vi "Open.vi"(8 "Error In":errorcluster, 10 "Username":string, 11 "Hostname / IP":string="localhost") -> (0 "Error Out":errorcluster, 3 "Hue Config":T1)   [LabVIEW 2020, in "LMH-Hue.lvlib"]
uses:
  LMH-Hue.lvlib
  Private/Type Defs/Hue Ref.ctl
  <vilib>/httpClient/ClientHandle.ctl
  Private/Type Defs/Light Data.ctl
  <vilib>/httpClient/LabVIEWHTTPClient.lvlib
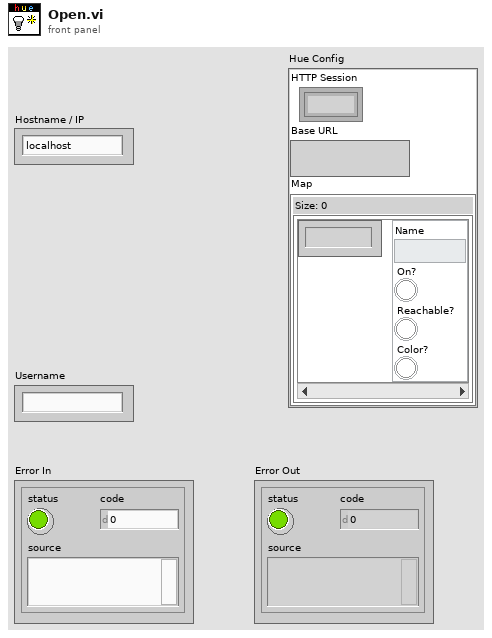
[diagram p1: front panel]
types:
  T1 = typedef "LMH-Hue.lvlib/Hue Ref.ctl" = cluster{"HTTP Session":T2, "Base URL":string, "Map":map{i32, T3}}
  T2 = typedef "LabVIEWHTTPClient.lvlib/ClientHandle.ctl" = refnum<k1>
  T3 = typedef "LMH-Hue.lvlib/Light Data.ctl" = cluster{"Name":string, "On?":bool, "Reachable?":bool, "Color?":bool}
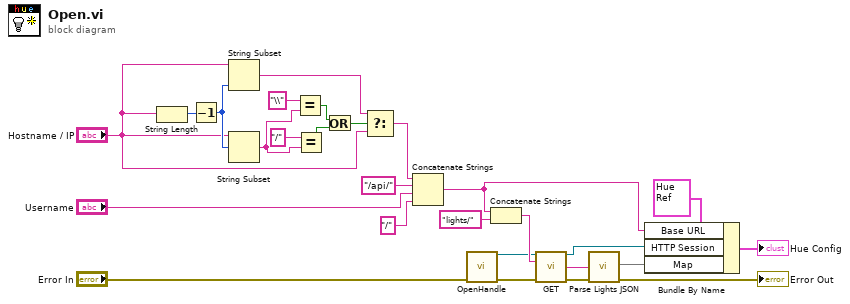
[diagram p0: block diagram]
diagram:
  n1 = String Length(string="Hostname / IP") -> (length=w26:i32)
  n2 = Decrement(x=w26) -> (x-1=w19:i32)
  n3 = String Subset(string="Hostname / IP", length (rest)=w19) -> (substring=w18:string)  [unwired: 1 in]
  n4 = String Subset(string="Hostname / IP", offset (0)=w19) -> (substring=w20:string)  [unwired: 1 in]
  n5 = Equal?(x="\\" ("y"), y=w20) -> (x = y?=w22:bool)
  n6 = Equal?(x="/" ("y"), y=w20) -> (x = y?=w24:bool)
  n7 = Or(x=w22, y=w24) -> (x .or. y?=w21:bool)
  n8 = Select(t=w18, s=w21, f="Hostname / IP") -> (s? t:f=w16:string)
  n9 = Concatenate Strings(w16, "/api/" ("string"), "Username", "/" ("string")) -> (w10:string)
  n10 = call <vilib>:"OpenHandle.vi"("error in (no error)"="Error In") -> ("client handle out"=w7:T2, "error out"=w5:errorcluster)  [unwired: 13 in]
  n11 = Concatenate Strings(w10, "lights/" ("string")) -> (w11:string)
  n12 = call <vilib>:"GET.vi"("client handle"=w7, "url"=w11, "error in (no error)"=w5) -> ("client handle out"=w6:T2, "body"=w4:string, "error out"=w3:errorcluster)  [unwired: 9 in, 1 out]
  n13 = call "Parse Lights JSON.vi"("error in"=w3, "Light JSON"=w4) -> ("error out"=→"Error Out":errorcluster, "Light Map"=w1:map{i32, T3})  [unwired: 8 in]
  n14 = Bundle By Name(cluster=T1 {"HTTP Session"=refnum, "Base URL"="", "Map"={}} ("Hue Config"), "Base URL"=w10, "HTTP Session"=w6, "Map"=w1) -> (→"Hue Config":T1)
